vi "escape for query.vi"(11 "String":string) -> (3 "String 2":string)   [LabVIEW 2011]
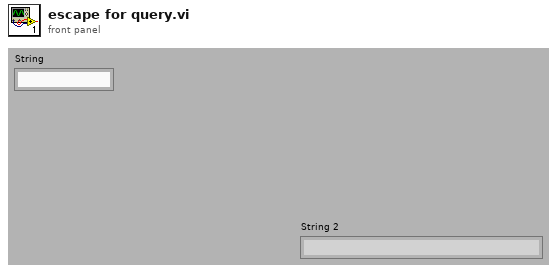
[diagram p1: front panel]
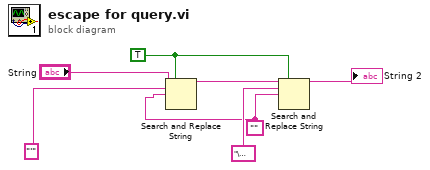
[diagram p0: block diagram]
diagram:
  w1 = ""
  w4 = TRUE ("replace all? (F)")
  n1 = Search and Replace String(replace all?=w4, input string="String", search string="'", replace string=w1) -> (result string=w5:string)  [unwired: 4 in, 3 out]
  n2 = Search and Replace String(replace all?=w4, input string=w5, search string="\u0000", replace string=w1) -> (result string=→"String 2":string)  [unwired: 4 in, 3 out]
